vi "FeedbackNodeDemo.vi"() -> ()   [LabVIEW 2018]
panel:
  out "Output":dbl
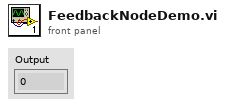
[diagram p1: front panel]
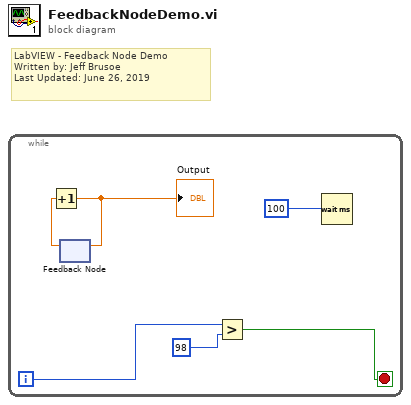
[diagram p0: block diagram]
diagram:
  # "LabVIEW - Feedback Node Demo\nWritten by: Jeff Brusoe\nLast Updated: June 26, 2019"
  n1 = while {
    i -> [w4]
    stop <- w2 stop-if-true
    n2 = feedback #1() -> (w6:dbl)  [unwired: 1 in]
    n3 = Increment(x=w6) -> (x+1=w5:dbl)
    "Output" <- w5
    n4 = feedback-in #1(w5) -> ()
    n5 = Greater?(x=w4, y=98 ("x")) -> (0:w2:bool)
    n6 = Wait (ms)(milliseconds to wait=u32 100 ("millisecond timer value")) -> ()  [unwired: 1 out]
  }
